vi "Run.vi"() -> ()   [LabVIEW 2016, in "DronaTest.lvlib"]
uses:
  DronaTest.lvlib
  <vilib>/addons/_JKI Toolkits/Caraya/run-tests/Run Test (LibraryRefnum).vi
  <vilib>/addons/_JKI Toolkits/Caraya/Caraya.lvlib
panel:
  out "error out":errorcluster
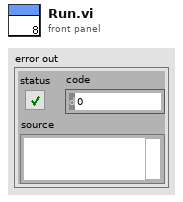
[diagram p1: front panel]
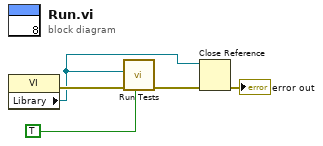
[diagram p0: block diagram]
diagram:
  n1 = property class="VI"() -> (error out=w5:errorcluster, "Library"=w2:refnum<vi>)  [unwired: 2 in, 1 out]
  n2 = call-poly <vilib>:"Run Tests.vi"("Verbose"=TRUE, "error in"=w5, "Library Refnum"=w2) -> ("error out"=w3:errorcluster)  [unwired: 7 in, 1 out]
  n3 = Close Reference(reference=w2, error in (no error)=w3) -> (error out=→"error out":errorcluster)
